vi "转换行结束符.vi"(9 "转换至":enum16{"CR", "LF", "CRLF"}(ring), 10 "输入字符串":string) -> (1 "输出字符串":string)   [LabVIEW 2012]
doc: "Converts all EOLs in the string to the type specified. A CRLF pair (\\r\\n) is considered to be one EOL. Therefore all CRLF pairs may be converted to just a CR or just a LF. Likewise single CRs or LFs may be converted to CRLF pairs. LabVIEW's Write File VIs have this option built into them, but Serial, TCP-IP, and others do not. There is no way to \"escape\" a CR, LF, or CRLF as not an EOL so be careful when using this utility."
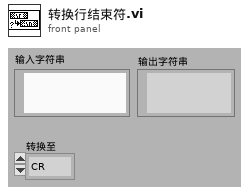
[diagram p1: front panel]
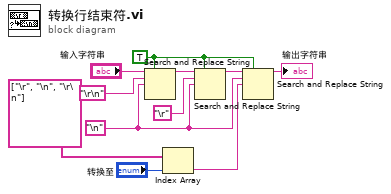
[diagram p0: block diagram]
diagram:
  w7 = TRUE ("replace all? (F)")
  w6 = "\n" ("search string")
  n1 = Search and Replace String(replace all?=w7, input string="输入字符串", search string="\r\n", replace string=w6) -> (result string=w10:string)  [unwired: 4 in, 3 out]
  n2 = Index Array(array=string[] ["\r", "\n", "\r\n"], index="转换至") -> (element=w3:string)
  n3 = Search and Replace String(replace all?=w7, input string=w10, search string="\r", replace string=w6) -> (result string=w8:string)  [unwired: 4 in, 3 out]
  n4 = Search and Replace String(replace all?=w7, input string=w8, search string=w6, replace string=w3) -> (result string=→"输出字符串":string)  [unwired: 4 in, 3 out]
